vi "RT Main.vi"() -> ()   [LabVIEW 2021]
uses:
  <vilib>/Platform/TimedLoop/XDataNode/timing_clust.ctl
  <vilib>/Platform/TimedLoop/XDataNode/nitl_modes.ctl
  <vilib>/Platform/TimedLoop/XDataNode/wakeup.ctl
  <vilib>/FPGAPlugInAG/myRIO-1900/niLvFpga_Open_myRIO-1900.vi
  <vilib>/rvi/interface/common/dynamic/niFpgaDynamicAddResources.vi
  <vilib>/Utility/error.llb/Error Cluster From Error Code.vi
  <vilib>/rvi/errors/niLvFpgaAdjustHostInterfaceError.vi
  <vilib>/FPGAPlugInAG/Dynamic/niLvFpga_Close_Dynamic.vi
  <vilib>/rvi/interface/nirviOpenFPGA/nirviOpenFPGA.xnode
  FPGA Bitfiles/lightstripprojec_FPGATarget_FPGAMain_V6m3OHc8nzM.lvbitx
  FPGA Main.vi
  <vilib>/Platform/TimedLoop/XDataNode/XDataNode.xnode
  <vilib>/rvi/interface/nirviMethod/nirviMethod.xnode
  <vilib>/rvi/interface/nirviCloseFPGA/nirviCloseFPGA.xnode
  <vilib>/Platform/TimedLoop/XDataNode/XDNodeRunTimeDep.lvlib
  <vilib>/rvi/errors/niLvFpgaMergeErrorWithErrorCode.vi
  <vilib>/FPGAPlugInAG/Dynamic/niLvFpga_WriteFifo_Dynamic.vi
  <vilib>/FPGAPlugInAG/Dynamic/niLvFpga_StopFifo_Dynamic.vi
panel:
  in  "Create":bool
  out "Iteration ms":i64=20
  in  "stop":bool
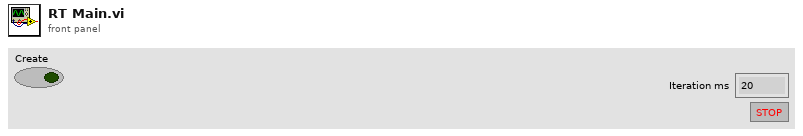
[diagram p1: front panel]
types:
  T1 = typedef "XDNodeRunTimeDep.lvlib/timing_clust.ctl" = cluster{"Expected End [f-1]":u64, "Actual End [f-1]":u64, "Finished Late? [f-1]":bool, "Expected End [i-1]":u64, "Actual End [i-1]":u64, "Finished Late? [i-1]":bool, "Expected Start [i]":u64, "Actual Start [i]":u64, "Expected Start [f]":u64, "Actual Start [f]":u64, "Source Name":string, "Structure Name":string, "Period":i64, "Deadline":i64, "Offset":i64, "Start":i64, "Priority":i32, "Timeout":i32, "Mode":T2, "Wakeup Reason":T3, "Error":errorcluster, "Source Type":string, "Secondary Source Type":string, "Global End Time":u64, "Global Start Time":u64, "Frame Duration":u64, "Iteration Duration":u64, "Assigned CPU":i32, "I/O Scan Engine Mode":u32}
  T2 = typedef "XDNodeRunTimeDep.lvlib/nitl_modes.ctl" = enum32{"No Change", "Process missed periods, maintain original phase", "Discard missed periods, maintain original phase", "Process missed periods, ignore original phase", "Discard missed periods, ignore original phase"}
  T3 = typedef "XDNodeRunTimeDep.lvlib/wakeup.ctl" = enum32{"Normal", "Aborted", "Asynchronous wakeup", "Timing source error", "Timed loop error", "Timeout"}
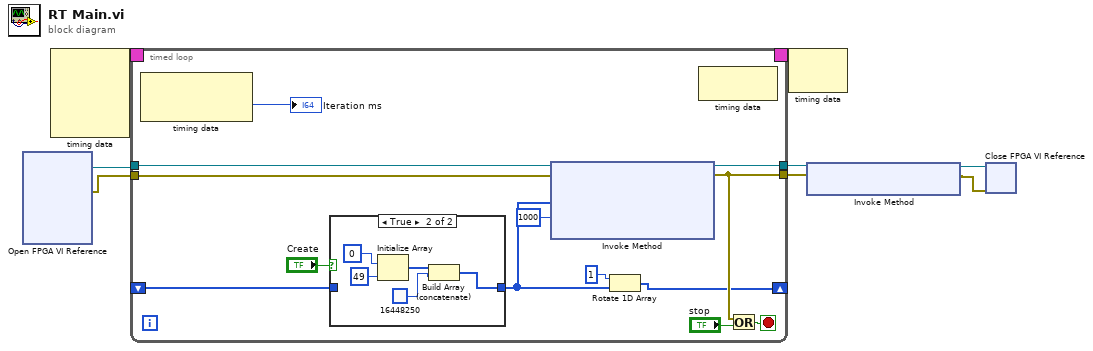
[diagram p0: block diagram]
diagram:
  n1 = xnode "Open FPGA VI Reference"() -> ("FPGA VI Reference Out"=w6:refnum<k20>, "error out"=w5:errorcluster)  [unwired: 2 in]
  n2 = node-c288() -> (w8:T1)  [unwired: 4 in]
  n3 = timed-loop {
    timing: w8 -> [_]
    timing-out: [_] -> w7
    tunnel: w6 -> [w20]
    tunnel: [w19] -> w4
    tunnel: [w17] -> w1
    shift-right: [w14] -> _
    shift-left: _ -> [w12]
    tunnel: w5 -> [w13]
    stop <- w18 stop-if-true
    n4 = node-c288() -> (→"Iteration ms":i64)  [unwired: 1 in, 1 out]
    n5 = case shown="True" "Create" {
      tunnel: [w22 w23] -> w11
      tunnel: w12 -> [w22 _]
      frame False {
      }
      frame True {
        n6 = Initialize Array(0 ("Color"), 49 ("dimension size")) -> (w25:i32[])
        n7 = Build Array (concatenate)(w25, u32 16448250) -> (w23:u32[])
      }
    }
    n8 = xnode "Invoke Method"("FPGA VI Reference In"=w20, "error in"=w13, "Data"=w11, "Timeout (ms)"=1000) -> ("FPGA VI Reference Out"=w19:refnum<k20>, "error out"=w17:errorcluster)  [unwired: 1 out]
    n9 = Rotate 1D Array(1:w11, 2:1 ("n")) -> (0:w14:u32[])
    n10 = node-c288() -> ()  [unwired: 1 in, 1 out]
    n11 = Or(x=w17, y="stop") -> (x .or. y?=w18:bool)
  }
  n12 = node-c288(w7) -> ()  [unwired: 1 out]
  n13 = xnode "Invoke Method"("FPGA VI Reference In"=w4, "error in"=w1) -> ("FPGA VI Reference Out"=w3:refnum<k20>, "error out"=w2:errorcluster)
  n14 = xnode "Close FPGA VI Reference"("FPGA VI Reference In"=w3, "error in"=w2) -> ()  [unwired: 1 out]
